vi "EPA aktiv genug Punkte.vi"(11 "Aktiv":T1) -> (2 "OK":bool, 3 "Aktiv out":T1)   [LabVIEW 2020, in "Linearisierung v2.lvlib"]
uses:
  Linearisierung v2.lvlib
  AktivArray.ctl
  AktivButton.ctl
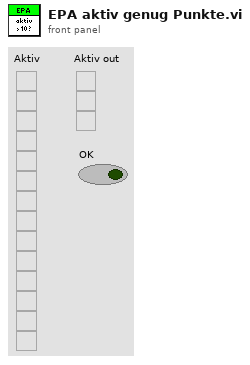
[diagram p1: front panel]
types:
  T1 = typedef "Linearisierung v2.lvlib/AktivArray.ctl" = T2[]
  T2 = typedef "Linearisierung v2.lvlib/AktivButton.ctl" = bool
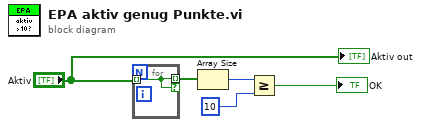
[diagram p0: block diagram]
diagram:
  n1 = for {
    tunnel: "Aktiv" -> [w6] mode=indexing
    tunnel: [w6] -> w2 mode=indexing if=w6
  }
  n2 = Array Size(array=w2) -> (size(s)=w3:i32)
  n3 = Greater Or Equal?(x=w3, y=10) -> (x >= y?=→"OK":bool)
  "Aktiv out" <- "Aktiv"
